vi "Unpack Latching Boolean Value Change.vi"(11 "LatchingBooleanValueChange In":refnum<class "LatchingBooleanValueChange.lvclass">) -> (2 "NewVal":bool, 3 "Control Label":string)   [LabVIEW 2015, in "LatchingBooleanValueChange.lvclass"]
uses:
  LatchingBooleanValueChange.lvclass
  LatchingBooleanValueChange.lvclass/LatchingBooleanValueChange.ctl
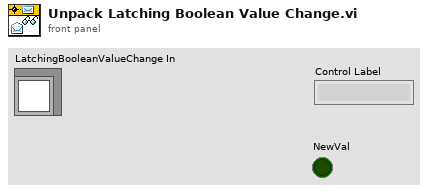
[diagram p1: front panel]
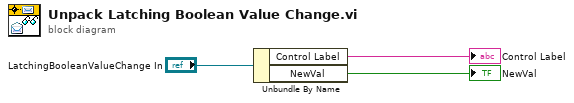
[diagram p0: block diagram]
diagram:
  n1 = Unbundle By Name("LatchingBooleanValueChange In") -> ("Control Label"=→"Control Label":string, "NewVal"=→"NewVal":bool)
